vi "GLB_Project.vi"() -> ()   [LabVIEW 2019]
panel:
  out "First Run Check":bool
  in  "Btn_Open":refnum<vi>
  in  "Project List":refnum<vi>
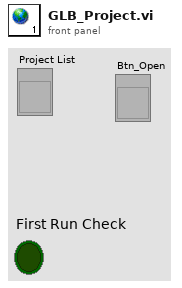
[diagram p1: front panel]
diagram:
